vi "json Parse Variant - string path.vi"(8 "error in (no error)":errorcluster, 9 "default":variant, 10 "path":string, 11 "JSON Document in":refnum<class "JSON Document.lvclass">) -> (0 "error out":errorcluster, 2 "value":variant, 3 "JSON Document out":refnum<class "JSON Document.lvclass">)   [LabVIEW 2015, in "JSON Document.lvclass"]
uses:
  JSON Document.lvclass
  JSON Document.lvclass/JSON Document.ctl
  rapidjson wrapper/rapidjson wrapper.lvlib
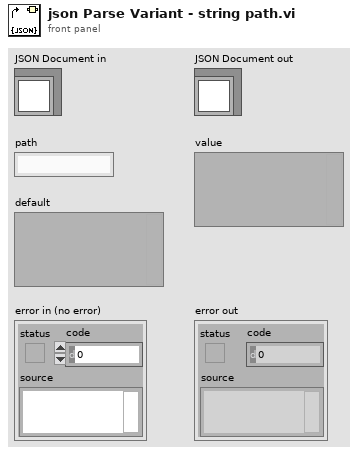
[diagram p1: front panel]
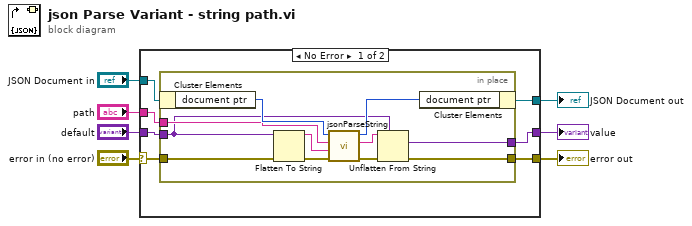
[diagram p0: block diagram]
diagram:
  n1 = case shown="No Error" "error in (no error)" {
    selector: "error in (no error)" -> [w11 w28]
    tunnel: [w10 w28] -> w6
    tunnel: [w9 w27] -> w4
    tunnel: "JSON Document in" -> [w14 w27]
    tunnel: "default" -> [w13 w26]
    tunnel: "path" -> [w12 _]
    tunnel: [w8 w26] -> w1
    frame No Error {
      n2 = in-place {
        in-place-border: w13 -> [w17]
        in-place-border: w12 -> [w23]
        in-place-border: w11 -> [w21]
        in-place-border: [w18] -> w10
        in-place-border: [w15] -> w8
        n3 = in-place-cluster #1(w14) -> ("document ptr"=w25:i64)
        n4 = Flatten To String(anything=w17, error in (no error)=w21) -> (data string=w22:string, error out=w20:errorcluster)  [unwired: 2 in, 1 out]
        n5 = call "jsonParseString.vi"("error in (no error)"=w20, "default"=w22, "path"=w23, "d in"=w25) -> ("error out"=w19:errorcluster, "value"=w16:string, "d out"=w24:i64)  [unwired: 5 in]
        n6 = Unflatten From String(type=w17, binary string=w16, error in (no error)=w19) -> (value=w15:variant, error out=w18:errorcluster)  [unwired: 2 in, 1 out]
        n7 = in-place-cluster #1("document ptr"=w24) -> (w9:refnum<class "JSON Document.lvclass">)
      }
    }
    frame Error {
    }
  }
  "error out" <- w6
  "JSON Document out" <- w4
  "value" <- w1
